vi "Check Scorer Availability.vi"(8 "error in (no error)":errorcluster, 10 "Submission":refnum<class "Submission.lvclass">, 11 "SOL-Server in":refnum<class "SOL-Server.lvclass">) -> (0 "error out":errorcluster, 3 "SOL-Server out":refnum<class "SOL-Server.lvclass">)   [LabVIEW 2020, in "Summer of LabVIEW.lvlib" / "SOL-Server.lvclass"]
uses:
  SOL-Server.lvclass
  Submission/Submission.lvclass
  SOL-Server.lvclass/SOL-Server.ctl
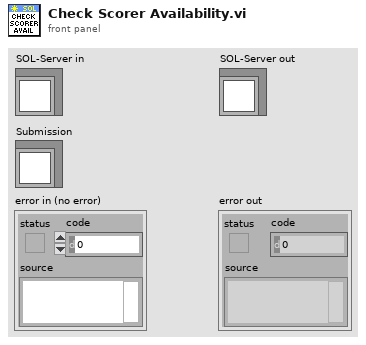
[diagram p1: front panel]
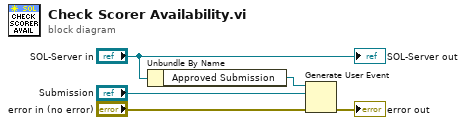
[diagram p0: block diagram]
diagram:
  n1 = Unbundle By Name("SOL-Server in") -> ("Approved Submission"=w4:refnum<user-event>)
  n2 = Generate User Event(user event=w4, event data cluster="Submission", error in="error in (no error)") -> (error out=→"error out":errorcluster)  [unwired: 1 in, 1 out]
  "SOL-Server out" <- "SOL-Server in"
